vi "S2C_PCIe7841_Proc_DigitalReadWrite.vi"(7 "Command":string, 8 "Error In":errorcluster, 11 "Data In":string) -> (0 "Error Out":errorcluster, 1 "ExpReply?":bool, 3 "Data Out":string)   [LabVIEW 2015]
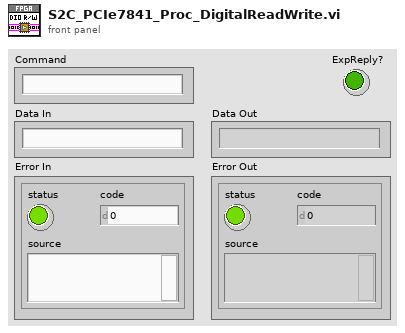
[diagram p1: front panel]
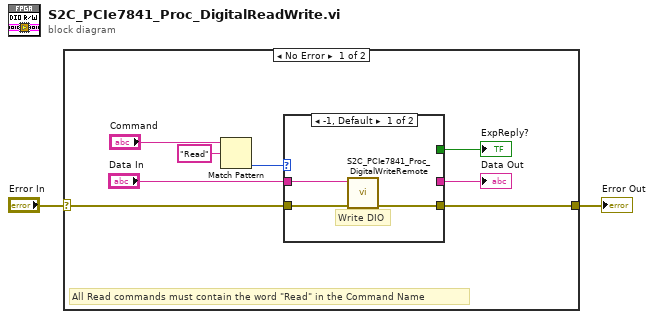
[diagram p0: block diagram]
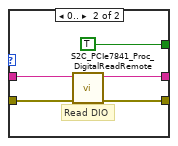
[diagram p2: hidden frame]
diagram:
  n1 = case shown="No Error" "Error In" {
    selector: "Error In" -> [w10 w19]
    tunnel: [w3 w19] -> w1
    frame No Error {
      # "All Read commands must contain the word \"Read\" in the Command Name"
      n2 = Match Pattern(string="Command", regular expression="Read") -> (offset past match=w7:i32)  [unwired: 1 in, 3 out]
      n3 = case shown="-1, Default" w7 {
        tunnel: w10 -> [w13 w18]
        tunnel: "Data In" -> [w12 w16]
        tunnel: [w11 w17] -> w3
        tunnel: [_ w15] -> w5
        tunnel: [_ TRUE] -> w4
        frame -1, Default {
          # "Write DIO"
          n4 = call "S2C_PCIe7841_Proc_DigitalWriteRemote.vi"("Error In"=w13, "Data"=w12) -> ("Error Out"=w11:errorcluster)  [unwired: 9 in]
        }
        frame 0.. {
          # "Read DIO"
          n5 = call "S2C_PCIe7841_Proc_DigitalReadRemote.vi"("Error In"=w18, "Data"=w16) -> ("Error Out"=w17:errorcluster, "State"=w15:string)  [unwired: 8 in]
        }
      }
      "Data Out" <- w5
      "ExpReply?" <- w4
    }
    frame Error {
    }
  }
  "Error Out" <- w1
